vi "Test Function 2.vi"(1 "x":refnum<class "Dual.lvclass">) -> (0 "f(x)":refnum<class "Dual.lvclass">)   [LabVIEW 2020, in "Tests.lvlib"]
uses:
  Tests.lvlib
  classes/Dual/Dual.lvclass
  classes/Dual/Dual.lvclass/Dual.ctl
  930c01a5-af24-4fc8-853d-8e8a583689cf.vi
  ace0f43f-1084-42ba-8d09-d9a18b478c7b.vi
  f48648b4-129d-4950-9652-f61e2f21534e.vi
  31379033-37d7-452c-bd52-dec53acfffcb.vi
  aaf71634-71ef-4bc3-b03a-9c7642836158.vi
  9ef6d408-8375-43dd-a8d9-eaccb68f813f.vi
  db240006-a983-41ee-8d48-78b54fd92577.vi
  c1017a04-84fc-4a4c-aa2c-b450438ee351.vi
  0fd89b59-dbab-4ddc-a326-d058eb74ff38.vi
  9675d4d4-ae23-477e-8d8f-3c0c97cc4d45.vi
  702ed0a6-02eb-46dc-b919-45e713aac3dd.vi
  e4211f5f-2c82-4891-87e2-c2d4c866cf83.vi
  265f0275-4443-4c76-87b6-9198b516cfb7.vi
  a4ace3d8-7dbc-4a5e-8e65-637f99b5b1f9.vi
  930c01a5-af24-4fc8-853d-8e8a583689cf.vi/5957e011-cf56-4527-b6ed-13c3a4ca997b.vi
  classes/Dual/Write a.vi
  ace0f43f-1084-42ba-8d09-d9a18b478c7b.vi/5957e011-cf56-4527-b6ed-13c3a4ca997b.vi
  f48648b4-129d-4950-9652-f61e2f21534e.vi/5957e011-cf56-4527-b6ed-13c3a4ca997b.vi
  31379033-37d7-452c-bd52-dec53acfffcb.vi/3c652a79-6380-41bc-942e-772f8e5d7896.vi
  classes/Dual/Read a and b.vi
  classes/Dual/Write a and b.vi
  aaf71634-71ef-4bc3-b03a-9c7642836158.vi/2c1e17fb-7848-4799-bd87-2ce00a1d4466.vi
  9ef6d408-8375-43dd-a8d9-eaccb68f813f.vi/957074e8-cc3b-4647-8ff1-d975a744cd4e.vi
  db240006-a983-41ee-8d48-78b54fd92577.vi/6ff4ae4f-abf9-4314-930a-0354c37082e1.vi
  c1017a04-84fc-4a4c-aa2c-b450438ee351.vi/b6499733-2759-4852-aa6b-3ec1516ef704.vi
  c1017a04-84fc-4a4c-aa2c-b450438ee351.vi/ce7907ec-4dc6-4618-8708-ad667a8e3a23.vi
  0fd89b59-dbab-4ddc-a326-d058eb74ff38.vi/968883c3-f1f3-473a-bfc5-8cde3e5b01f7.vi
  0fd89b59-dbab-4ddc-a326-d058eb74ff38.vi/bec82738-76c0-439a-a1c7-54fdd631a6e8.vi
  9675d4d4-ae23-477e-8d8f-3c0c97cc4d45.vi/cbb88b8f-dcf9-42b8-ac98-84298073c153.vi
  702ed0a6-02eb-46dc-b919-45e713aac3dd.vi/957074e8-cc3b-4647-8ff1-d975a744cd4e.vi
  e4211f5f-2c82-4891-87e2-c2d4c866cf83.vi/6101d903-ff9f-41ff-96b8-b42400c258cc.vi
  e4211f5f-2c82-4891-87e2-c2d4c866cf83.vi/5aba97ba-e1f8-4e08-94e3-f0ae7cb31178.vi
  265f0275-4443-4c76-87b6-9198b516cfb7.vi/6101d903-ff9f-41ff-96b8-b42400c258cc.vi
  265f0275-4443-4c76-87b6-9198b516cfb7.vi/5aba97ba-e1f8-4e08-94e3-f0ae7cb31178.vi
  a4ace3d8-7dbc-4a5e-8e65-637f99b5b1f9.vi/6101d903-ff9f-41ff-96b8-b42400c258cc.vi
  a4ace3d8-7dbc-4a5e-8e65-637f99b5b1f9.vi/5aba97ba-e1f8-4e08-94e3-f0ae7cb31178.vi
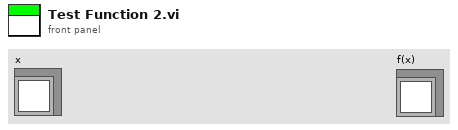
[diagram p1: front panel]
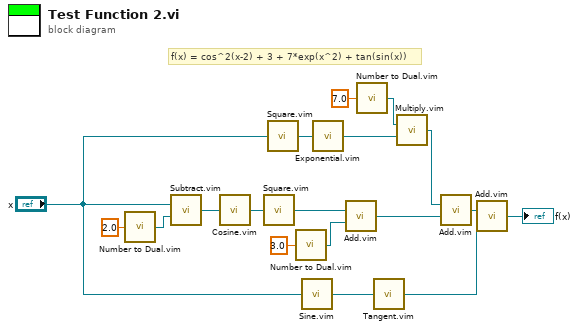
[diagram p0: block diagram]
diagram:
  # "f(x) = cos^2(x-2) + 3 + 7*exp(x^2) + tan(sin(x))"
  n1 = call "Number to Dual.vim"("Number"=2.0 ("a")) -> ("Dual"=w12:refnum<class "Dual.lvclass">)
  n2 = call "Subtract.vim"("x"="x", "y"=w12) -> ("x - y"=w11:refnum<class "Dual.lvclass">)  [unwired: 13 in]
  n3 = call "Cosine.vim"("x"=w11) -> ("cos(x)"=w14:refnum<class "Dual.lvclass">)
  n4 = call "Square.vim"("x"=w14) -> ("x^2"=w18:refnum<class "Dual.lvclass">)
  n5 = call "Square.vim"("x"="x") -> ("x^2"=w9:refnum<class "Dual.lvclass">)
  n6 = call "Number to Dual.vim"("Number"=3.0 ("a")) -> ("Dual"=w15:refnum<class "Dual.lvclass">)
  n7 = call "Sine.vim"("x"="x") -> ("sin(x)"=w3:refnum<class "Dual.lvclass">)
  n8 = call "Exponential.vim"("x"=w9) -> ("exp(x)"=w8:refnum<class "Dual.lvclass">)
  n9 = call "Add.vim"("x"=w18, "y"=w15) -> ("x + y"=w10:refnum<class "Dual.lvclass">)  [unwired: 13 in]
  n10 = call "Number to Dual.vim"("Number"=7.0 ("a")) -> ("Dual"=w6:refnum<class "Dual.lvclass">)
  n11 = call "Tangent.vim"("x"=w3) -> ("tan(x)"=w2:refnum<class "Dual.lvclass">)
  n12 = call "Multiply.vim"("x"=w6, "y"=w8) -> ("x * y"=w5:refnum<class "Dual.lvclass">)  [unwired: 13 in]
  n13 = call "Add.vim"("x"=w5, "y"=w10) -> ("x + y"=w4:refnum<class "Dual.lvclass">)  [unwired: 13 in]
  n14 = call "Add.vim"("x"=w4, "y"=w2) -> ("x + y"=→"f(x)":refnum<class "Dual.lvclass">)  [unwired: 13 in]
